vi "BPCS-Malicious-DE-OnePID-User-Event.vi"() -> ()   [LabVIEW 2018]
uses:
  <vilib>/Platform/TimedLoop/XDataNode/timing_clust.ctl
  <vilib>/Platform/TimedLoop/XDataNode/nitl_modes.ctl
  <vilib>/Platform/TimedLoop/XDataNode/wakeup.ctl
  <vilib>/addons/control/pid/pid.llb/PID Advanced (DBL).vi
  <vilib>/Platform/TimedLoop/XDataNode/XDataNode.xnode
  <vilib>/Platform/TimedLoop/XDataNode/XDNodeRunTimeDep.lvlib
  <vilib>/addons/control/pid/NI_PID_pid.lvlib
panel:
  out "PID Output":dbl format="%.2f"
  out "error out":errorcluster
  out "element":dbl
  out "Finished Late? [i-1]":bool
  out "Actual End [i-1]":i64
  out "Expected End [i-1]":i64
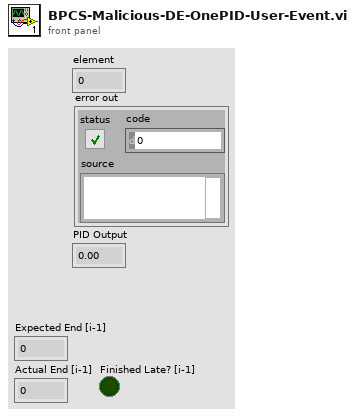
[diagram p1: front panel]
types:
  T1 = typedef "XDNodeRunTimeDep.lvlib/timing_clust.ctl" = cluster{"Expected End [f-1]":u64, "Actual End [f-1]":u64, "Finished Late? [f-1]":bool, "Expected End [i-1]":u64, "Actual End [i-1]":u64, "Finished Late? [i-1]":bool, "Expected Start [i]":u64, "Actual Start [i]":u64, "Expected Start [f]":u64, "Actual Start [f]":u64, "Source Name":string, "Structure Name":string, "Period":i64, "Deadline":i64, "Offset":i64, "Start":i64, "Priority":i32, "Timeout":i32, "Mode":T2, "Wakeup Reason":T3, "Error":errorcluster, "Source Type":string, "Secondary Source Type":string, "Global End Time":u64, "Global Start Time":u64, "Frame Duration":u64, "Iteration Duration":u64, "Assigned CPU":i32, "I/O Scan Engine Mode":u32}
  T2 = typedef "XDNodeRunTimeDep.lvlib/nitl_modes.ctl" = enum32{"No Change", "Process missed periods, maintain original phase", "Discard missed periods, maintain original phase", "Process missed periods, ignore original phase", "Discard missed periods, ignore original phase"}
  T3 = typedef "XDNodeRunTimeDep.lvlib/wakeup.ctl" = enum32{"Normal", "Aborted", "Asynchronous wakeup", "Timing source error", "Timed loop error", "Timeout"}
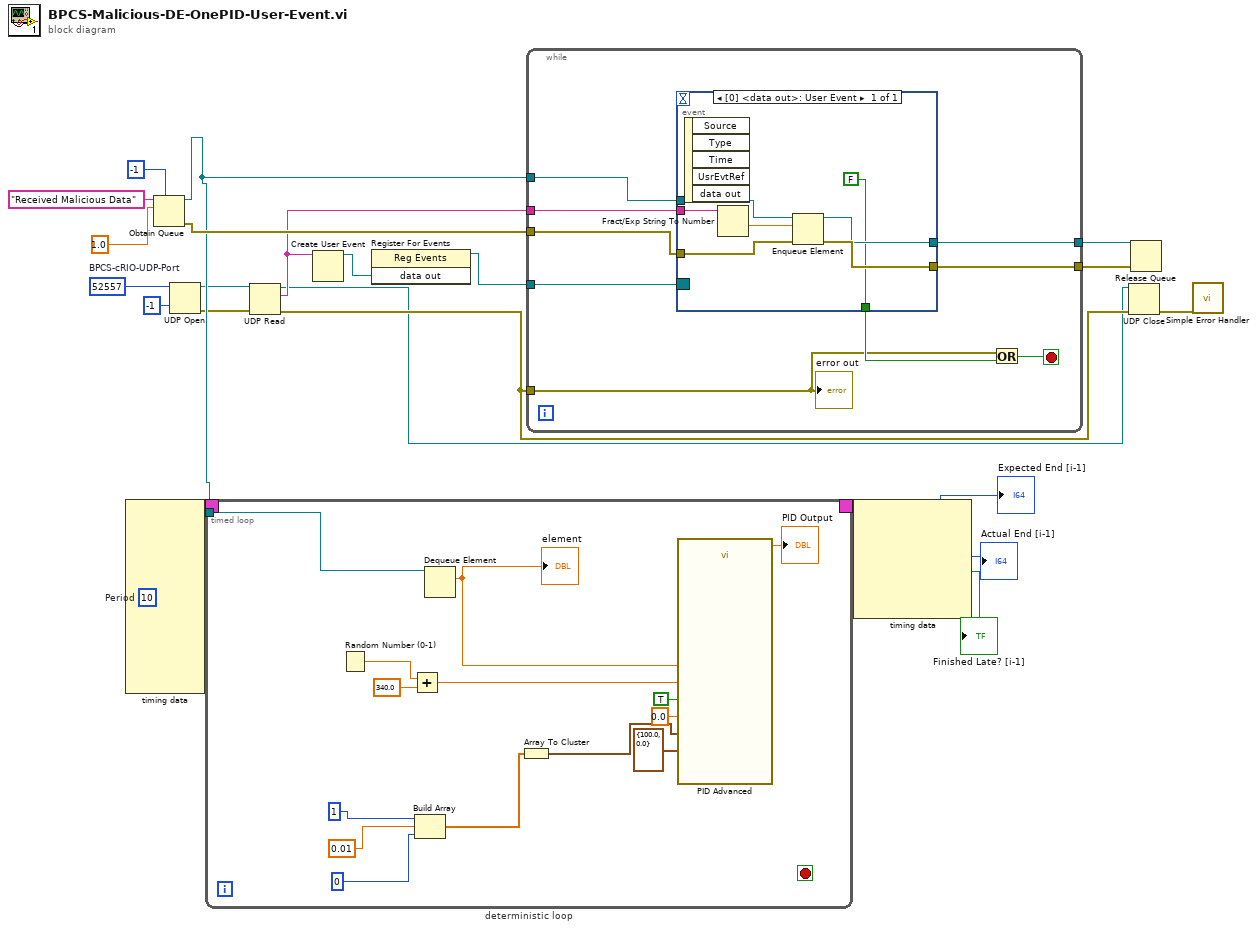
[diagram p0: block diagram]
diagram:
  w12 = i64 10  # Period
  w23 = u16 52557  # BPCS-cRIO-UDP-Port
  n1 = node-c288 ("Input Node")(w12) -> (w14:T1)  [unwired: 9 in]
  n2 = Obtain Queue(max queue size (-1, unlimited)=-1, name (unnamed)="Received Malicious Data", element data type=1.0) -> (queue out=w8:refnum<queue>, error out=w15:errorcluster)  [unwired: 2 in, 1 out]
  n3 = UDP Open(9:-1 ("timeout ms (25000)"), 11:w23) -> (port=w6:refnum<k16>, 0:w7:errorcluster)  [unwired: 3 in, 1 out]
  n4 = timed-loop "deterministic loop" {
    timing: w14 -> [_]
    timing-out: [_] -> w13
    tunnel: w8 -> [w25]
    stop <- _ stop-if-true
    n5 = Random Number (0-1)() -> (number: 0 to 1=w29:dbl)
    n6 = Add(x=w29, y=340.0) -> (x+y=w27:dbl)
    n7 = Build Array(1, 0.01, 0) -> (w33:dbl[])
    n8 = Dequeue Element(queue=w25) -> (element=w24:dbl)  [unwired: 2 in, 3 out]
    "element" <- w24
    n9 = Array To Cluster(array=w33) -> (cluster=w32:cluster{"[0]":dbl, "[1]":dbl, "[2]":dbl})
    n10 = call-poly <vilib>:"PID Advanced.vi"("setpoint"=w24, "output range"=cluster{"output high":dbl, "output low":dbl} {"output high"=100.0, "output low"=0.0}, "auto? (T)"=TRUE, "manual control"=0.0, "process variable"=w27, "PID gains"=w32) -> ("output"=→"PID Output":dbl)  [unwired: 8 in, 1 out]
  }
  n11 = UDP Read(connection ID=w6, 8:w7) -> (data out=w4:string, error out=w5:errorcluster, 3:w3:refnum<k16>)  [unwired: 1 in, 3 out]
  n12 = Create User Event(user event datatype=w4) -> (user event=w2:refnum<user-event>)  [unwired: 1 in, 1 out]
  n13 = register-events(w2) -> (reference out=w1:refnum<event-registration>)  [unwired: 2 in, 1 out]
  n14 = while {
    tunnel: [w47] -> w17
    tunnel: [w46] -> w16
    tunnel: w8 -> [w43]
    tunnel: w15 -> [w45]
    tunnel: w5 -> [w42]
    tunnel: w4 -> [w41]
    tunnel: w1 -> [w40]
    stop <- w48 stop-if-true
    n15 = event shown="[0] <data out>: User Event" {
      selector: w40 -> [_]
      dyn-events: _ -> [_]
      timeout: _ -> [_]
      tunnel: [w54] -> w47
      tunnel: [w53] -> w46
      tunnel: w43 -> [w52]
      tunnel: w45 -> [w51]
      tunnel: [FALSE] -> w44
      tunnel: w41 -> [w49]
      event User Event {
        n16 = event-data() -> ()  [unwired: 1 in, 5 out]
        n17 = Fract/Exp String To Number(string=w49) -> (number=w55:dbl)  [unwired: 3 in, 1 out]
        n18 = Enqueue Element(queue=w52, element=w55, error in (no error)=w51) -> (queue out=w53:refnum<queue>, error out=w54:errorcluster)  [unwired: 1 in, 1 out]
      }
    }
    n19 = Or(x=w42, y=w44) -> (x .or. y?=w48:bool)
    "error out" <- w42
  }
  n20 = node-c288 ("Output Node")(w13) -> (→"Expected End [i-1]":i64, →"Actual End [i-1]":i64, →"Finished Late? [i-1]":bool)  [unwired: 3 out]
  n21 = UDP Close(connection ID=w3, 8:w5) -> (error out=w22:errorcluster)  [unwired: 1 out]
  n22 = Release Queue(queue=w16, error in (no error)=w17) -> ()  [unwired: 1 in, 3 out]
  n23 = call <vilib>:"Simple Error Handler.vi"("error in (no error)"=w22) -> ()  [unwired: 4 in, 5 out]
